vi "Write AxisNumber.vi"(8 "error in (no error)":errorcluster, 10 "AxisNumber":u8, 11 "StopMovement Msg in":refnum<class "StopMovement Msg.lvclass">) -> (0 "error out":errorcluster, 3 "StopMovement Msg out":refnum<class "StopMovement Msg.lvclass">)   [LabVIEW 2015, in "CS++Motor.lvlib" / "StopMovement Msg.lvclass"]
uses:
  StopMovement Msg.lvclass
  StopMovement Msg.lvclass/StopMovement Msg.ctl
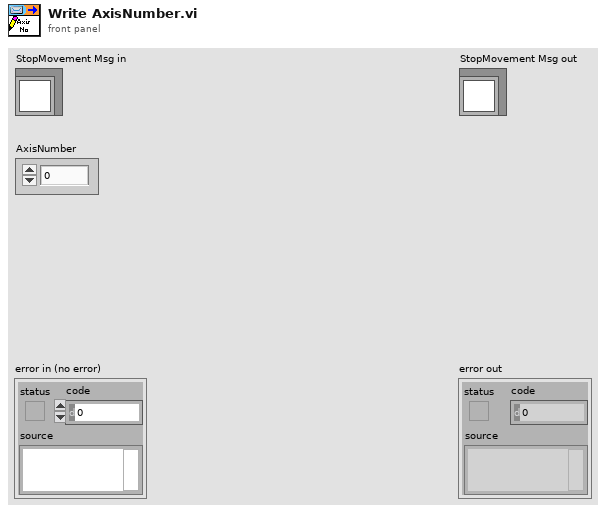
[diagram p1: front panel]
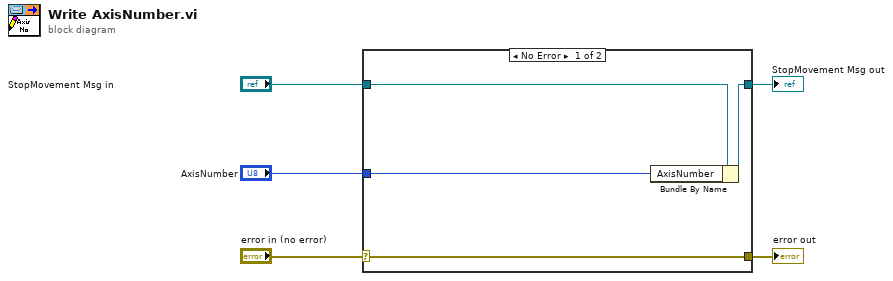
[diagram p0: block diagram]
diagram:
  n1 = case shown="No Error" "error in (no error)" {
    selector: "error in (no error)" -> [w9 w10]
    tunnel: [w9 w10] -> w4
    tunnel: [w7 w11] -> w2
    tunnel: "StopMovement Msg in" -> [w8 w11]
    tunnel: "AxisNumber" -> [w6 _]
    frame No Error {
      n2 = Bundle By Name(cluster=w8, "AxisNumber"=w6) -> (w7:refnum<class "StopMovement Msg.lvclass">)
    }
    frame Error {
    }
  }
  "error out" <- w4
  "StopMovement Msg out" <- w2
